vi "Subvi in range.vi"(8 "max":u16, 9 "Input":u16) -> (0 "Overflow":bool, 1 "Underflow":bool)   [LabVIEW 2017]
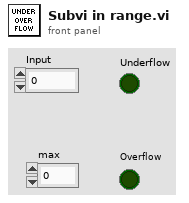
[diagram p1: front panel]
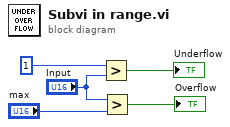
[diagram p0: block diagram]
diagram:
  n1 = Greater?(x=u16 1 ("min"), y="Input") -> (0:→"Underflow":bool)
  n2 = Greater?(x="Input", y="max") -> (0:→"Overflow":bool)
